vi "Pull HW Data for Plots.vi"(8 "error in (no error)":errorcluster) -> (0 "IMOvl":bool, 1 "IMPeakPower":dbl[](array[numeric]), 2 "IMPower":dbl[](array[numeric]) format="%.2f", 3 "IMFreqs":dbl[](array[numeric]) format="%.2f", 4 "error out":errorcluster)   [LabVIEW 2011]
uses:
  API/Controls/PIM.API.Command.Unique.ctl
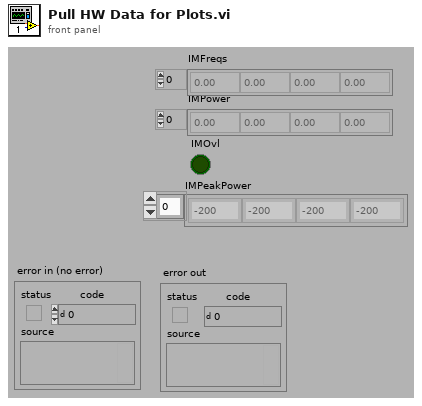
[diagram p1: front panel]
types:
  T1 = typedef "PIM.API.Command.Unique.ctl" = cluster{"#attributes":cluster{"Action":string}, "Double":dbl[], "Integer":i32[], "Boolean":bool[], "String":string[]}
  T2 = typedef "PIM.API.Response.Unique.ctl" = cluster{"#attributes":cluster{"Action":string, "Units":string}, "Double":dbl[], "Integer":i32[], "Boolean":bool[], "String":string[], "Sample":T3[], "Status":cluster{"#attributes":cluster{"Error":bool, "Code":i32}, "Message":string}[]}
  T3 = typedef "PIM.API.Response.Samples.ctl" = cluster{"TX1":cluster{"#attributes":cluster{"Frequency":dbl, "Power_dBm":dbl, "Power_Watts":dbl, "CheckTx":bool, "Unleveled":bool, "Squelched":bool, "Temperature":dbl, "ToneOn":bool}}, "TX2":cluster{"#attributes":cluster{"Frequency":dbl, "Power_dBm":dbl, "Power_Watts":dbl, "CheckTx":bool, "Unleveled":bool, "Squelched":bool, "Temperature":dbl, "ToneOn":bool}}, "IM":cluster{"#attributes":cluster{"Frequency":dbl, "Power_dBm":dbl, "PeakPower_dBm":dbl, "Power_dBc":dbl, "PeakPower_dBc":dbl, "IM_Order":u8, "IM Overload":bool}}[], "#attributes":cluster{"Count":u32, "Total":u32, "Finished?":bool, "Sweep Leg":T4, "F1":dbl, "F2":dbl, "FStep":dbl}}
  T4 = typedef "iQA Sweep Behavior.ctl" = enum16{"F2Down", "F1Up", "RxMultiIM"}
  T5 = cluster{"#attributes":cluster{"Error":bool, "Code":i32}, "Message":string}[]
  T6 = cluster{"#attributes":cluster{"Error":bool, "Code":i32}, "Message":string}
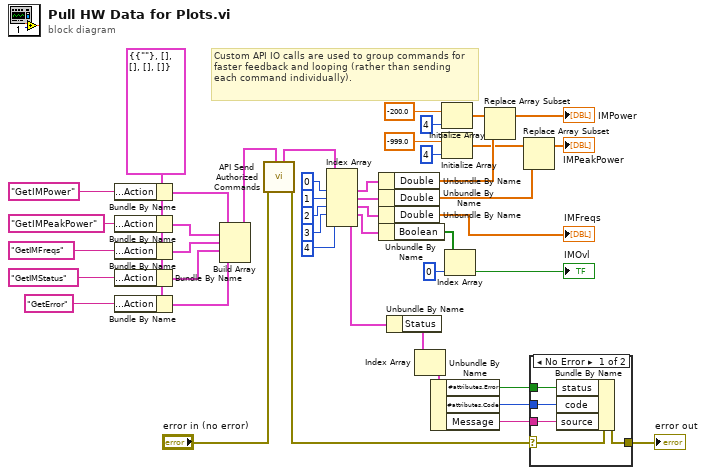
[diagram p0: block diagram]
diagram:
  w23 = T1 {"#attributes"={"Action"=""}, "Double"=[], "Integer"=[], "Boolean"=[], "String"=[]}
  # "Custom API IO calls are used to group commands for faster feedback and looping (rather than sending each command individually)."
  n1 = Bundle By Name(cluster=w23, "#attributes.Action"="GetIMPower") -> (w44:T1)
  n2 = Bundle By Name(cluster=w23, "#attributes.Action"="GetIMPeakPower") -> (w43:T1)
  n3 = Bundle By Name(cluster=w23, "#attributes.Action"="GetIMFreqs") -> (w42:T1)
  n4 = Bundle By Name(cluster=w23, "#attributes.Action"="GetIMStatus") -> (w41:T1)
  n5 = Bundle By Name(cluster=w23, "#attributes.Action"="GetError") -> (w22:T1)
  n6 = Build Array(w44, w43, w42, w41, w22) -> (w1:T1[])
  n7 = call "API Send Authorized Commands.vi"("Commands"=w1, "error in (no error)"="error in (no error)") -> ("error out"=w16:errorcluster, "Responses"=w2:T2[])  [unwired: 7 in, 1 out]
  n8 = Index Array(array=w2, index #1=0 ("index"), index #2=1 ("index"), index #3=2 ("index"), index #4=3 ("index"), index #5=4 ("index")) -> (element #1=w32:T2, element #2=w36:T2, element #3=w35:T2, element #4=w37:T2, element #5=w14:T2)
  n9 = Unbundle By Name(w32) -> ("Double"=w7:dbl[])
  n10 = Unbundle By Name(w36) -> ("Double"=w5:dbl[])
  n11 = Unbundle By Name(w35) -> ("Double"=→"IMFreqs":dbl[])
  n12 = Unbundle By Name(w37) -> ("Boolean"=w26:bool[])
  n13 = Unbundle By Name(w14) -> ("Status"=w17:T5)
  n14 = Index Array(array=w17) -> (element=w18:T6)  [unwired: 1 in]
  n15 = Unbundle By Name(w18) -> ("#attributes.Error"=w19:bool, "#attributes.Code"=w20:i32, "Message"=w21:string)
  n16 = Initialize Array(-200.0, 4 ("dimension size")) -> (w8:dbl[])
  n17 = Initialize Array(-999.0, 4 ("dimension size")) -> (w6:dbl[])
  n18 = Index Array(array=w26, index=0) -> (element=→"IMOvl":bool)
  n19 = Replace Array Subset(array=w8, new element=w7) -> (→"IMPower":dbl[])  [unwired: 1 in]
  n20 = Replace Array Subset(array=w6, new element=w5) -> (→"IMPeakPower":dbl[])  [unwired: 1 in]
  n21 = case shown="No Error" w16 {
    selector: w16 -> [w46 w51]
    tunnel: w19 -> [w50 _]
    tunnel: w20 -> [w49 _]
    tunnel: w21 -> [w48 _]
    tunnel: [w47 w51] -> w13
    frame No Error {
      n22 = Bundle By Name(cluster=w46, "status"=w50, "code"=w49, "source"=w48) -> (w47:errorcluster)
    }
    frame Error {
    }
  }
  "error out" <- w13
